vi "config.vi"(8 "error in (no error)":errorcluster, 10 "ZTAAC Configuration":T2={"Config Dir"=path "/home/ttsai/Documents/stash/ts_tcs_ofc/configData", "Inst Name"=enum."lsst", "OptStateEsti Config File Name"="pinv.esti", "Mapping File Name"="sensorNameToFieldIdx.txt", "Wavelength Table"="effWaveLength.txt", "Intrinc Zk File Name"="intrinsic_zn", "y2 Corection File Name"="y2.txt", "Index DOF File Name"="idxDOF.txt", "OptCtrl Config File Name"="optiPSSN_x00.ctrl", "State 0 File Name"="state0inDof.txt", "Weighting File Name"="imgQualWgt.txt", "PSSN Alpha File Name"="pssn_alpha.txt", "Authority Files"={"Rigid Body Stroke File"="rbStroke.txt", "M1M3 Subsystem"={"Mirror"="M1M3", "Actuatro Force File"="M1M3_1um_156_force.txt"}, "M2 Subsystem"={"Mirror"="M2", "Actuatro Force File"="M2_1um_force.DAT"}, "Num of Bending Mode"=20}, "Sensor Id to Name File Name"="sensorIdToName.txt", "Truncation Threshold"=0.0001, "Default Gain"=0.7, "FWHM Threshold (arcsec)"=0.2}, 11 "ZTAAC in":refnum<class "ZTAAC.lvclass">) -> (0 "error out":errorcluster, 3 "ZTAAC out":refnum<class "ZTAAC.lvclass">)   [LabVIEW 2016, in "OfcFunc.lvlib" / "ZTAAC.lvclass"]
doc: "Do the configuration of Zernike to actuator adjustment calculator (ZTAAC). This is a high-level class to use the \"optical state estimator\" and \"optimal control\"."
uses:
  ZTAAC.lvclass
  StrictDef/InstName.ctl
  ZTAAC.lvclass/ZTAAC.ctl
  OptStateEsti/OptStateEsti.lvclass
  OptCtrl/OptCtrl.lvclass
  OfcFunc.lvlib
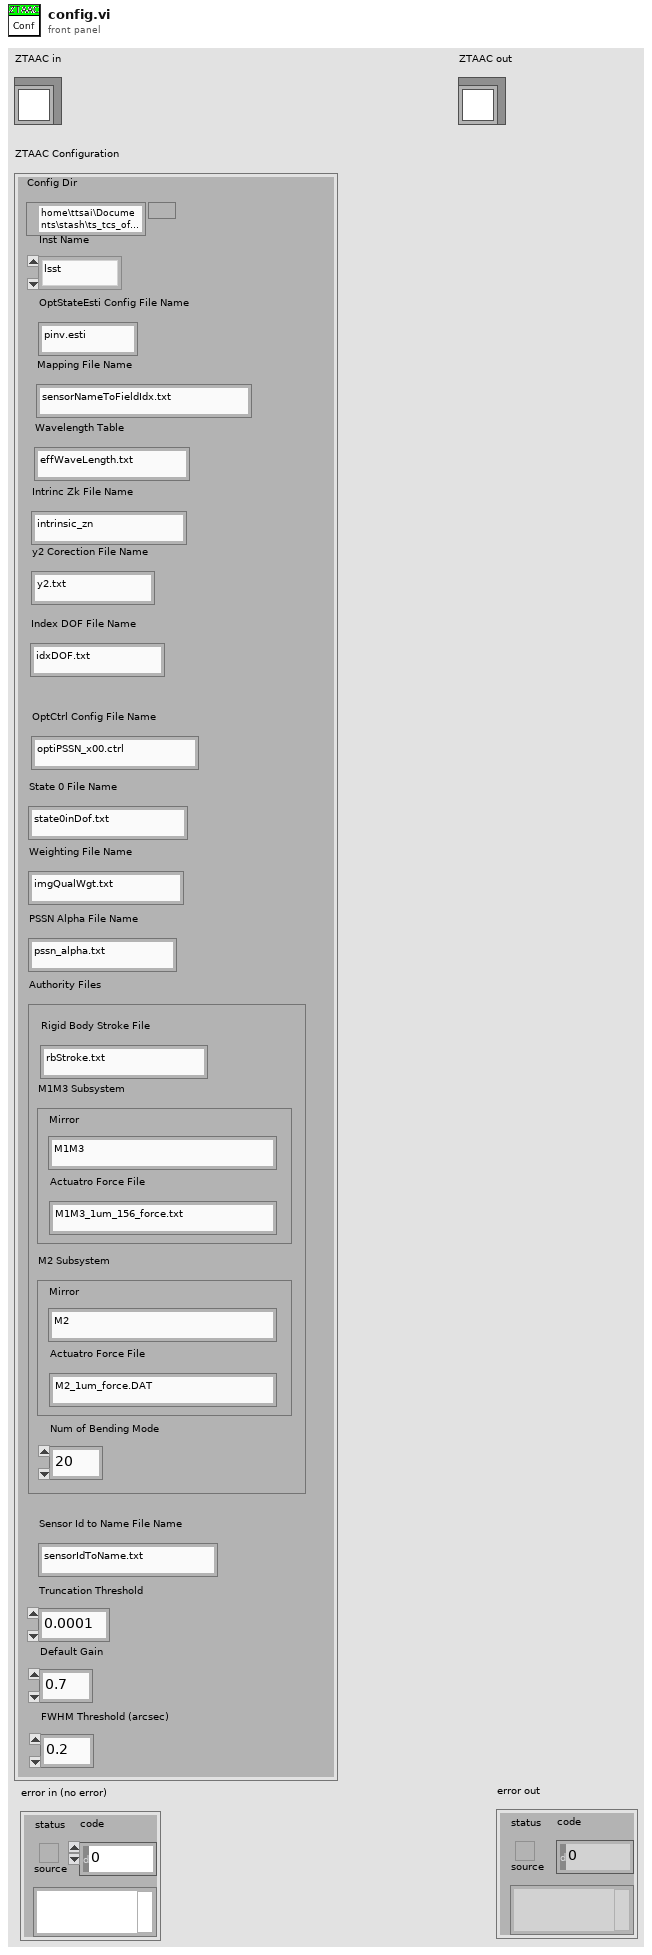
[diagram p1: front panel]
types:
  T1 = typedef "OfcFunc.lvlib/InstName.ctl" = enum16{"lsst", "comcam"}
  T2 = cluster{"Config Dir":path, "Inst Name":T1, "OptStateEsti Config File Name":string, "Mapping File Name":string, "Wavelength Table":string, "Intrinc Zk File Name":string, "y2 Corection File Name":string, "Index DOF File Name":string, "OptCtrl Config File Name":string, "State 0 File Name":string, "Weighting File Name":string, "PSSN Alpha File Name":string, "Authority Files":cluster{"Rigid Body Stroke File":string, "M1M3 Subsystem":cluster{"Mirror":string, "Actuatro Force File":string}, "M2 Subsystem":cluster{"Mirror":string, "Actuatro Force File":string}, "Num of Bending Mode":i32}, "Sensor Id to Name File Name":string, "Truncation Threshold":dbl, "Default Gain":dbl, "FWHM Threshold (arcsec)":dbl}
  T3 = cluster{"Rigid Body Stroke File":string, "M1M3 Subsystem":cluster{"Mirror":string, "Actuatro Force File":string}, "M2 Subsystem":cluster{"Mirror":string, "Actuatro Force File":string}, "Num of Bending Mode":i32}
  T4 = cluster{"Config Dir":path, "Inst Name":T1, "OptStateEsti Config File Name":string, "Mapping File Name":string, "Wavelength Table":string, "Intrinc Zk File Name":string, "y2 Corection File Name":string, "Index DOF File Name":string}
  T5 = cluster{"Config Dir":path, "OptCtrl Config File Name":string, "Inst Name":T1, "State 0 File Name":string, "Weighting File Name":string, "PSSN Alpha File Name":string, "Authority Files":cluster{"Rigid Body Stroke File":string, "M1M3 Subsystem":cluster{"Mirror":string, "Actuatro Force File":string}, "M2 Subsystem":cluster{"Mirror":string, "Actuatro Force File":string}, "Num of Bending Mode":i32}}
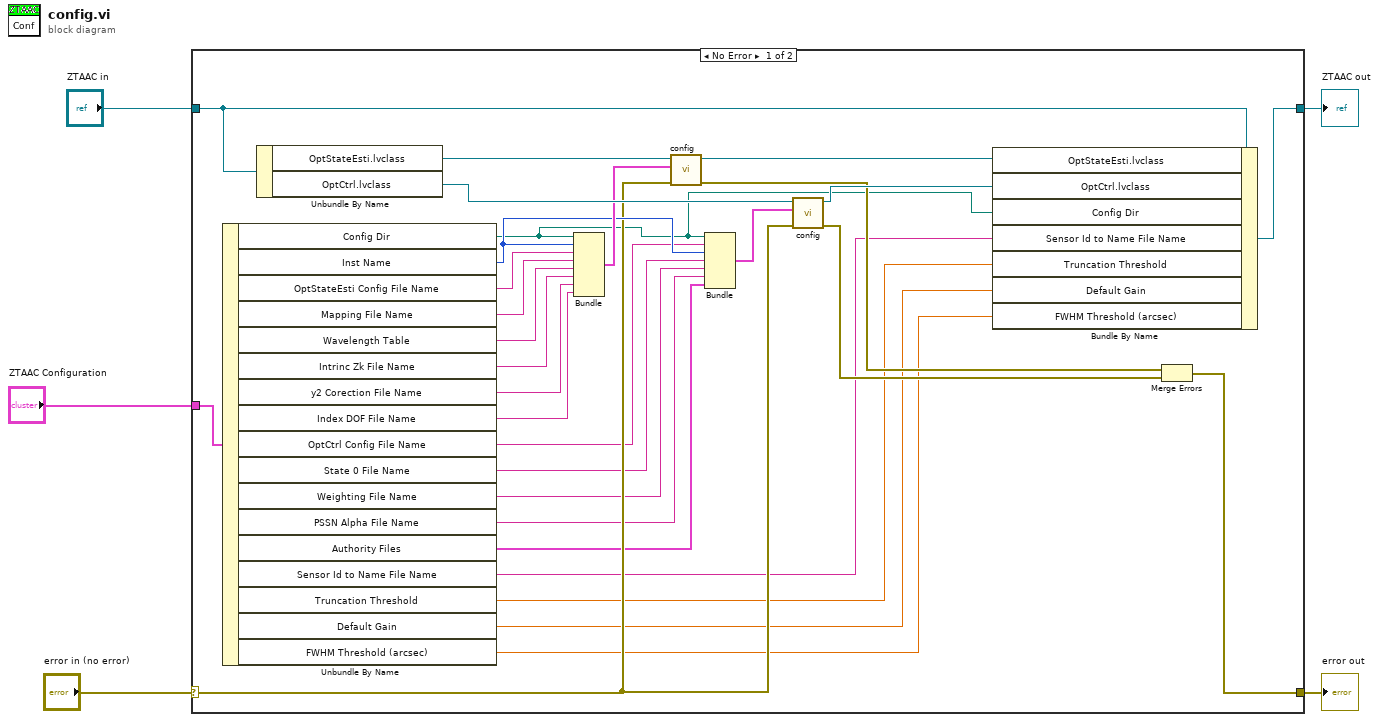
[diagram p0: block diagram]
diagram:
  n1 = case shown="No Error" "error in (no error)" {
    selector: "error in (no error)" -> [w20 w37]
    tunnel: [w17 w37] -> w4
    tunnel: [w23 w36] -> w2
    tunnel: "ZTAAC in" -> [w24 w36]
    tunnel: "ZTAAC Configuration" -> [w35 _]
    frame No Error {
      n2 = Unbundle By Name(w35) -> ("Config Dir"=w10:path, "Inst Name"=w26:T1, "OptStateEsti Config File Name"=w32:string, "Mapping File Name"=w31:string, "Wavelength Table"=w30:string, "Intrinc Zk File Name"=w29:string, "y2 Corection File Name"=w28:string, "Index DOF File Name"=w11:string, "OptCtrl Config File Name"=w12:string, "State 0 File Name"=w13:string, "Weighting File Name"=w14:string, "PSSN Alpha File Name"=w15:string, "Authority Files"=w16:T3, "Sensor Id to Name File Name"=w8:string, "Truncation Threshold"=w9:dbl, "Default Gain"=w7:dbl, "FWHM Threshold (arcsec)"=w6:dbl)
      n3 = Unbundle By Name(w24) -> ("OptStateEsti.lvclass"=w33:refnum<class "OptStateEsti.lvclass">, "OptCtrl.lvclass"=w34:refnum<class "OptCtrl.lvclass">)
      n4 = Bundle("Config Dir"=w10, "Inst Name"=w26, "OptStateEsti Config File Name"=w32, "Mapping File Name"=w31, "Wavelength Table"=w30, "Intrinc Zk File Name"=w29, "y2 Corection File Name"=w28, "Index DOF File Name"=w11) -> (w27:T4)  [unwired: 1 in]
      n5 = call "config.vi"("error in (no error)"=w20, "Configuration"=w27, "OptStateEsti in"=w33) -> ("error out"=w19:errorcluster, "OptStateEsti out"=w22:refnum<class "OptStateEsti.lvclass">)  [unwired: 7 in]
      n6 = Bundle("Config Dir"=w10, "OptCtrl Config File Name"=w12, "Inst Name"=w26, "State 0 File Name"=w13, "Weighting File Name"=w14, "PSSN Alpha File Name"=w15, "Authority Files"=w16) -> (w25:T5)  [unwired: 1 in]
      n7 = call "config.vi"("error in (no error)"=w20, "Configuration"=w25, "OptCtrl in"=w34) -> ("error out"=w18:errorcluster, "OptCtrl out"=w21:refnum<class "OptCtrl.lvclass">)  [unwired: 7 in]
      n8 = Bundle By Name(cluster=w24, "OptStateEsti.lvclass"=w22, "OptCtrl.lvclass"=w21, "Config Dir"=w10, "Sensor Id to Name File Name"=w8, "Truncation Threshold"=w9, "Default Gain"=w7, "FWHM Threshold (arcsec)"=w6) -> (w23:refnum<class "ZTAAC.lvclass">)
      n9 = Merge Errors(w19, w18) -> (w17:errorcluster)
    }
    frame Error {
    }
  }
  "error out" <- w4
  "ZTAAC out" <- w2
